vi "Keysight Counter.vi"(1 "Action":T4=enum."Identify", 2 "Parameters":variant) -> (6 "Output":variant, 7 "Stop":bool)   [LabVIEW 2025]
doc: "Author: Scott Hannahs <sth@magnet.fsu.edu>\n\nThis software is licensed for use under the “MIT License\"\nCopyright (c) 2025 Scott Hannahs, sth@sth@magnet.sthnet.net\n\nPermission is hereby granted, free of charge, to any person obtaining a copy of this software and associated documentation files (the \"Software\"), to deal in the Software without restriction, including without limitation the rights to use, copy, modify, merge, publish, distribute, sublicense, and/or sell copies of the Software, and to permit persons to whom the Software is furnished to do so, subject to the following conditions: The above copyright notice and this permission notice shall be included in all copies or substantial portions of the Software.\n\nTHE SOFTWARE IS PROVIDED \"AS IS\", WITHOUT WARRANTY OF ANY KIND, EXPRESS OR IMPLIED, INCLUDING BUT NOT LIMITED TO THE WARRANTIES OF MERCHANTABILITY, FITNESS FOR A PARTICULAR PURPOSE AND NONINFRINGEMENT. IN NO EVENT SHALL THE AUTHORS OR COPYRIGHT HOLDERS BE LIABLE FOR ANY CLAIM, DAMAGES OR OTHER LIABILITY, WHETHER IN AN ACTION OF CONTRACT, TORT OR OTHERWISE, ARISING FROM, OUT OF OR IN CONNECTION WITH THE SOFTWARE OR THE USE OR OTHER DEALINGS IN THE SOFTWARE."
uses:
  Sub Controls/Instrument Actions.ctl
  Sub Controls/Public.ctl
  Sub Controls/Instrument Match.ctl
  SubVIs/Counter Avg Control.ctl
  Sub Controls/Scan Output.ctl
  Sub Controls/Instrument IDN.ctl
  Sub Controls/User Event Command.ctl
panel:
  in  "Averaging":T1
  in  "Factory Reset":bool
  out "Title":string="Stanford Research Lockin"
  in  "VISA resource name":refnum<visa-resource-name>
  in  "Instruments":T2[](array[typedef])=[{"Model"="53230A", "Manufacturer"="Agilent Technologies", "Term Character"="", "Wait Time (mS)"=0, "Wait for SRQ"=FALSE, "Type"="Counter"}]
  out "Model":string
  in  "Address":u16(ring)
  in  "Public":T3
  out "Measurement":dbl[](array[numeric]) format="%^.3e"
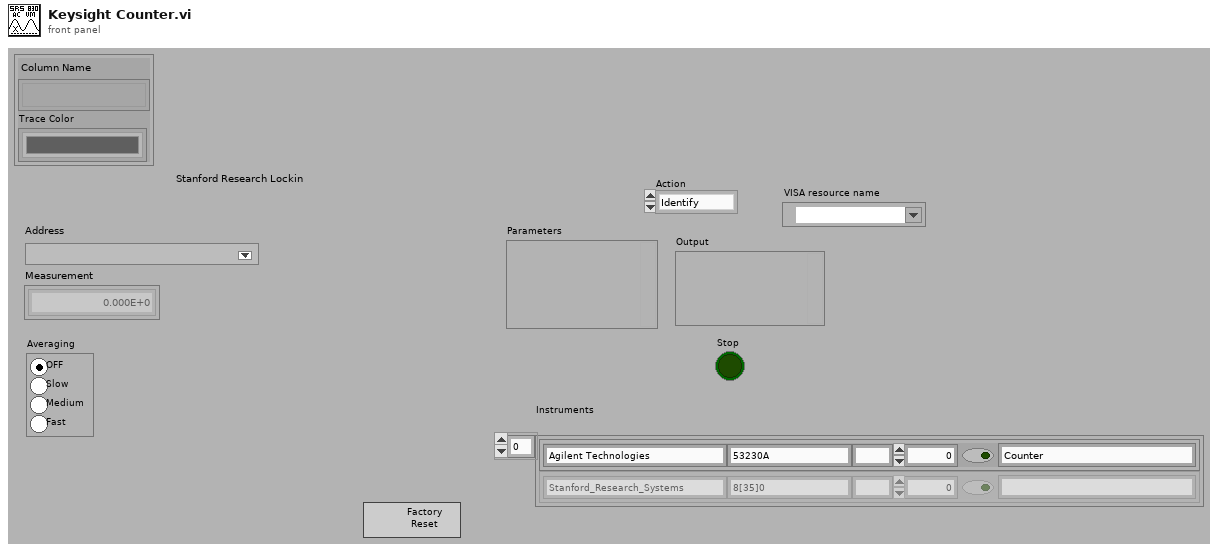
[diagram p1: front panel]
types:
  T1 = typedef "Counter Avg Control.ctl" = enum32{"Off", "Slow", "Medium", "Fast"}
  T2 = typedef "Instrument Match.ctl" = cluster{"Model":string, "Manufacturer":string, "Term Character":string, "Wait Time (mS)":u32, "Wait for SRQ":bool, "Type":string}
  T3 = typedef "Public.ctl" = cluster{"Column Name":string[], "Trace Color":u32[]}
  T4 = typedef "Instrument Actions.ctl" = enum16{"Scan", "Identify", "New", "Configure", "Initialize", "Test", "Read", "Close"}
  T5 = typedef "Scan Output.ctl" = cluster{"Manufacturer":string, "Model":string, "Info":string, "Revision":string, "error out":errorcluster}
  T6 = typedef "Instrument IDN.ctl" = cluster{"VISA Address":string, "Status":u16, "Manufacturer":string, "Model":string, "Info":string, "Info 2":string, "Misc Data":variant}
  T7 = typedef "User Event Command.ctl" = enum32{"Stop Config"}
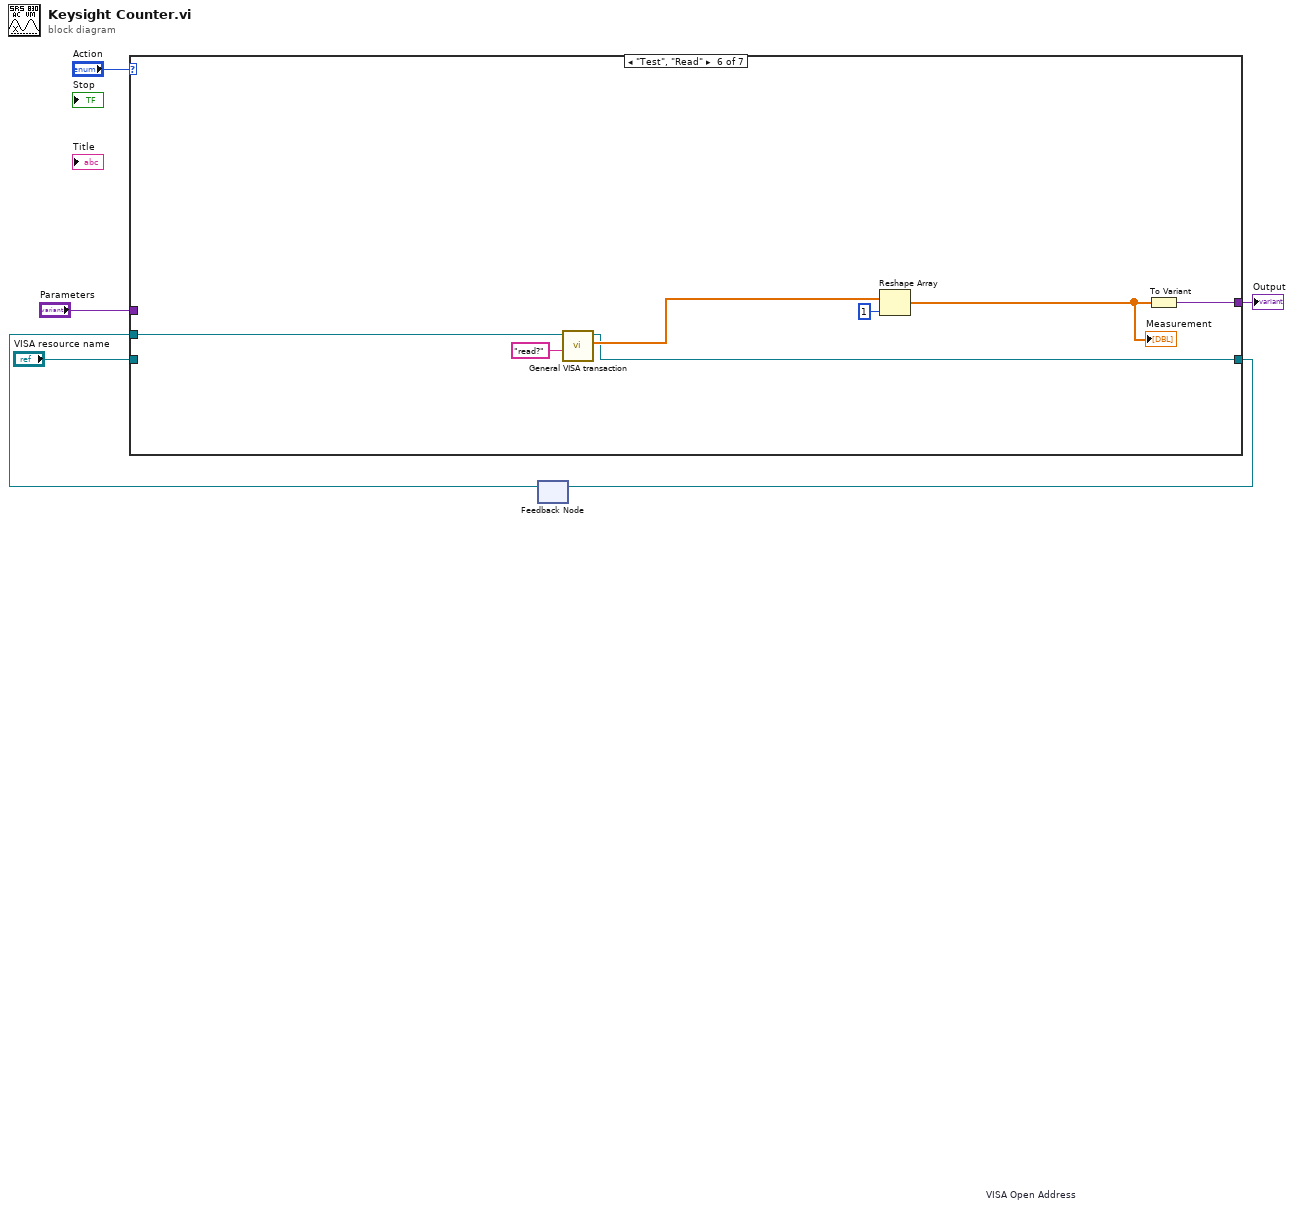
[diagram p0: block diagram]
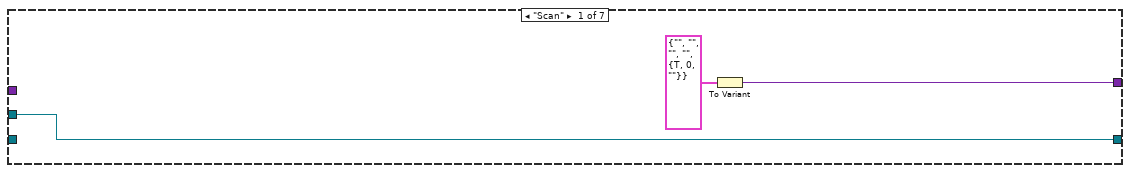
[diagram p2: hidden frame]
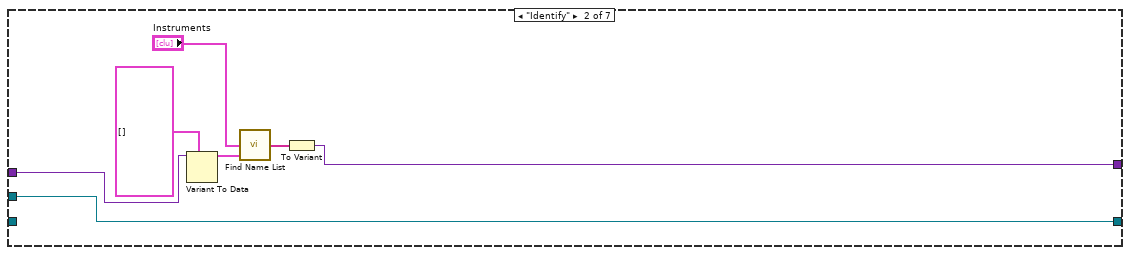
[diagram p3: hidden frame]
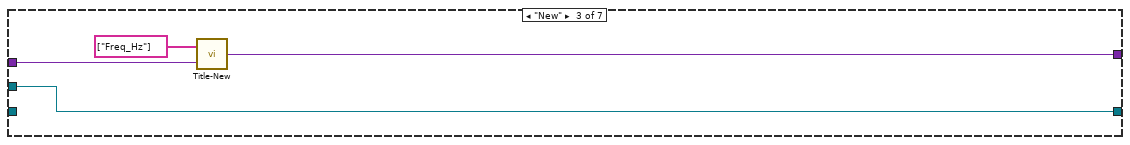
[diagram p4: hidden frame]
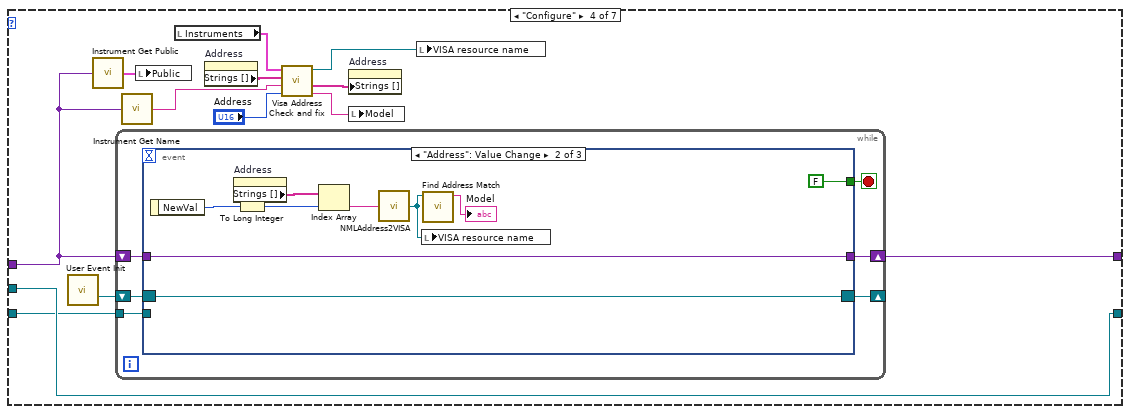
[diagram p5: hidden frame]
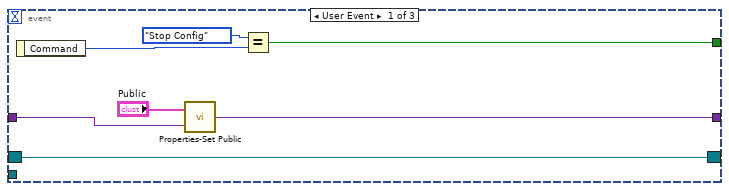
[diagram p6: hidden frame]
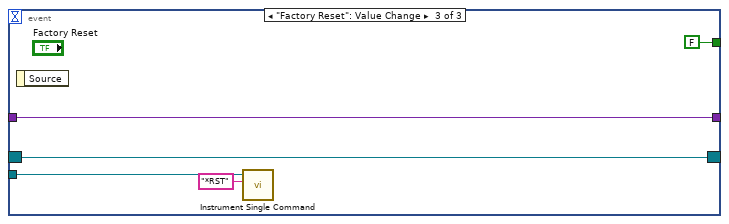
[diagram p7: hidden frame]
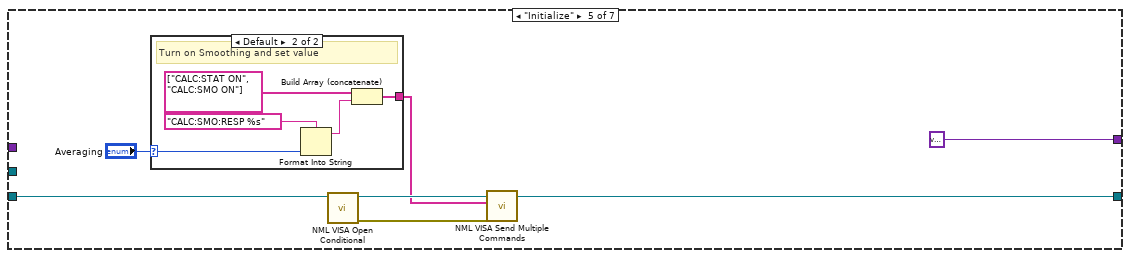
[diagram p8: hidden frame]
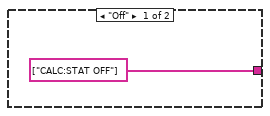
[diagram p9: hidden frame]
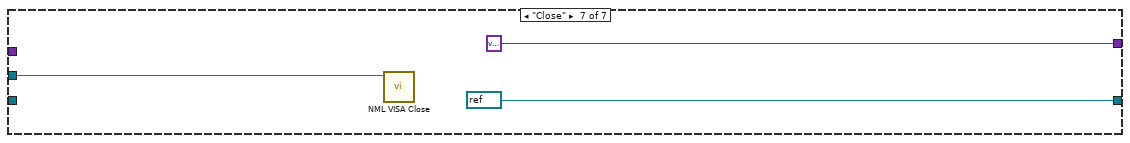
[diagram p10: hidden frame]
diagram:
  n1 = feedback #1 "VISA Open Address"() -> (w2:refnum<visa-resource-name>)  [unwired: 1 in]
  n2 = case shown="\"Test\", \"Read\"" "Action" {
    tunnel: [w8 w16 w19 w22 w64 w76 refnum<visa-resource-name> refnum ("Open VISA Resource name")] -> w3
    tunnel: w2 -> [w8 w16 w19 w22 _ w77 w81]
    tunnel: "Parameters" -> [_ w13 w20 w26 _ _ _]
    tunnel: [w7 w15 w17 w33 variant ("Variant") w80 variant ("Variant")] -> w5
    tunnel: "VISA resource name" -> [_ _ _ w21 w66 _ _]
    frame "Scan" {
      n3 = To Variant(anything=T5 {"Manufacturer"="", "Model"="", "Info"="", "Revision"="", "error out"={"status"=TRUE, "code"=0, "source"=""}} ("Scan Output")) -> (Variant=w7:variant)
    }
    frame "Identify" {
      n4 = Variant To Data(type=T6[] [], Variant=w13) -> (data=w11:T6[])  [unwired: 1 in, 1 out]
      n5 = call "Find Name List.vi"("Bus Scan"=w11, "Instruments"="Instruments") -> ("Names"=w10:string[])  [unwired: 1 in]
      n6 = To Variant(anything=w10) -> (Variant=w15:variant)
    }
    frame "New" {
      n7 = call "Title-New.vi"("Parameters"=w20, "Array"=string[] ["Freq_Hz"]) -> ("Instrument Prop"=w17:variant)
    }
    frame "Configure" {
      n8 = call "User Event Init.vi"() -> ("Event Registration Refnum"=w31:refnum<event-registration>)  [unwired: 14 in, 1 out]
      n9 = call "Instrument Get Public.vi"("Variant"=w26) -> ("Public"=w32:T3)
      n10 = while {
        shift-right: [w39] -> w33
        shift-left: w26 -> [w38]
        shift-right: [w35] -> _
        shift-left: w31 -> [w36]
        tunnel: w21 -> [w34]
        stop <- w37 stop-if-true
        n11 = event shown="[1] \"Address\": Value Change" {
          selector: w36 -> [w40 w55 w58]
          dyn-events: [w40 w55 w58] -> w35
          timeout: _ -> [_ _ _]
          tunnel: [w42 FALSE FALSE] -> w37
          tunnel: w38 -> [w45 w49 w59]
          tunnel: [w46 w49 w59] -> w39
          tunnel: w34 -> [_ _ w57]
          event User Event {
            n12 = event-data() -> ("Command"=w44:T7)  [unwired: 1 in]
            n13 = call "Properties-Set Public.vi"("Variant"=w45, "New Public"="Public") -> ("Variant 2"=w46:variant)
            n14 = Equal?(x=User_Event_Command."Stop Config", y=w44) -> (x = y?=w42:bool)
          }
          event "Address": Value Change {
            n15 = event-data() -> ("NewVal"=w53:u16)  [unwired: 1 in]
            n16 = property on="Address" class="Ring (strict)"() -> ("Strings []"=w52:string[])  [unwired: 2 in, 2 out]
            n17 = To Long Integer(number=w53) -> (32bit integer=w47:i32)
            n18 = Index Array(array=w52, index=w47) -> (element=w51:string)
            n19 = call "NMLAddress2VISA.vi"("NML Address"=w51) -> ("VISA resource name"=w48:refnum<visa-resource-name>)
            n20 = local write "VISA resource name"(w48) -> ()
            n21 = call "Find Address Match.vi"("VISA resource name"=w48) -> ("Model"=→"Model":string)  [unwired: 3 in, 3 out]
          }
          event "Factory Reset": Value Change {
            n22 = event-data() -> ()  [unwired: 1 in, 1 out]
            n23 = call "Instrument Single Command.vi"("Reset Command"="*RST", "VISA Name"=w57) -> ()  [unwired: 9 in, 1 out]
          }
        }
      }
      n24 = call "Instrument Get Name.vi"("Parameters"=w26) -> ("Type"=w27:string)
      n25 = local write "Public"(w32) -> ()
      n26 = local read "Instruments"() -> (w25:T2[])
      n27 = property on="Address" class="Ring (strict)"() -> ("Strings []"=w29:string[])  [unwired: 2 in, 2 out]
      n28 = call "Visa Address Check and fix.vi"("Instruments"=w25, "NML Addresses"=w29, "Name"=w27, "Address"="Address") -> ("VISA resource name"=w28:refnum<visa-resource-name>, "NML Addresses"=w24:string[], "Model"=w23:string)  [unwired: 4 out]
      n29 = property on="Address" class="Ring (strict)"("Strings []"=w24) -> ()  [unwired: 2 in, 2 out]
      n30 = local write "Model"(w23) -> ()
      n31 = local write "VISA resource name"(w28) -> ()
    }
    frame "Initialize" {
      n32 = case shown="Default" "Averaging" {
        selector: "Averaging" -> [_ w72]
        tunnel: [string[] ["CALC:STAT OFF"] w69] -> w62
        frame "Off" {
        }
        frame Default {
          # "Turn on Smoothing and set value"
          n33 = Format Into String(format string="CALC:SMO:RESP %s", w72) -> (resulting string=w71:string)  [unwired: 2 in, 1 out]
          n34 = Build Array (concatenate)(string[] ["CALC:STAT ON", "CALC:SMO ON"], w71) -> (w69:string[])
        }
      }
      n35 = call "NML VISA Open Conditional.vi"("VISA resource name"=w66) -> ("error out"=w61:errorcluster, "dup VISA Session"=w65:refnum<visa-resource-name>)  [unwired: 8 in, 1 out]
      n36 = call "NML VISA Send Multiple Commands.vi"("error in (no error)"=w61, "Commands"=w62, "VISA resource name"=w65) -> ("VISA resource name"=w64:refnum<visa-resource-name>)  [unwired: 8 in]
    }
    frame "Test", "Read" {
      n37 = call "General VISA transaction.vi"("Command String"="read?", "VISA Session"=w77) -> ("Measurement"=w79:dbl[], "dup VISA Session"=w76:refnum<visa-resource-name>)  [unwired: 4 in, 4 out]
      n38 = Reshape Array(w79, 1 ("dimension size")) -> (w78:dbl[])
      "Measurement" <- w78
      n39 = To Variant(anything=w78) -> (Variant=w80:variant)
    }
    frame "Close" {
      n40 = call "NML VISA Close.vi"("VISA resource name"=w81) -> ()  [unwired: 10 in, 1 out]
    }
  }
  "Output" <- w5
  n41 = feedback-in #1(w3) -> ()
